vi "Test_LIMS.vi"() -> ()   [LabVIEW 2019]
uses:
  TypeDef/Test.ctl
  TypeDef/Asset.ctl
  TypeDef/Step.ctl
  TypeDef/UpdateLimsTestStepData.ctl
  ByteGSAPIBase.lvclass
panel:
  out "Result Step 2":T1
  in  "instruction_automation":string
  in  "link_automation":string="https://bytelabs.sharepoint.com/:i:/r/sites/RD/Documenti%20condivisi/Knowledge/yoann-siloine-dyaxQ-aoGWY-unsplash.jpg?csf=1&web=1&e=iVCiSf"
  out "Result Step":T2
  in  "duration_hours":dbl
  in  "value":dbl
  in  "step index":i32
  in  "test index":i32
  out "Test Steps List":T3[](array[typedef])
  out "error out":errorcluster
  out "Tests for bench":T5[](array[typedef])
  in  "Postazione/Data":T6
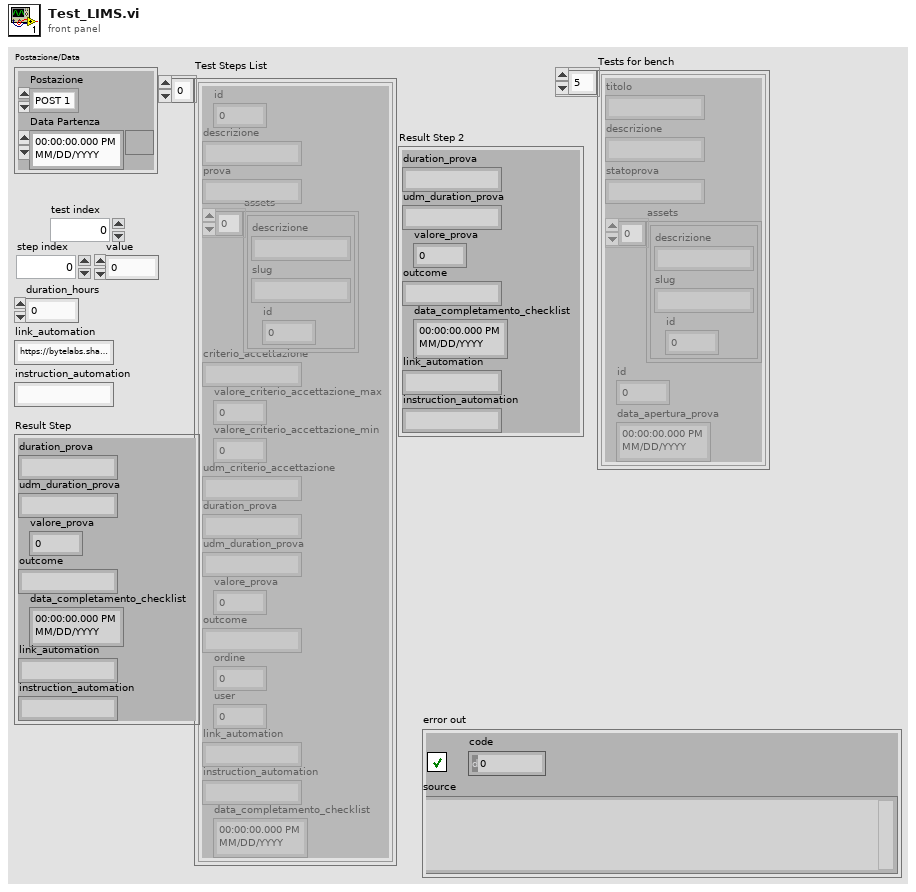
[diagram p1: front panel]
types:
  T1 = typedef "UpdateLimsTestStepData.ctl" = cluster{"duration_prova":string, "udm_duration_prova":string, "valore_prova":dbl, "outcome":string, "data_completamento_checklist":timestamp, "link_automation":string, "instruction_automation":string}
  T2 = cluster{"duration_prova":string, "udm_duration_prova":string, "valore_prova":dbl, "outcome":string, "data_completamento_checklist":timestamp, "link_automation":string, "instruction_automation":string}
  T3 = typedef "ByteGSWebAPI.lvlib/ByteGSAPIBase.lvclass/Step.ctl" = cluster{"id":i32, "descrizione":string, "prova":string, "assets":T4[], "criterio_accettazione":string, "valore_criterio_accettazione_max":dbl, "valore_criterio_accettazione_min":dbl, "udm_criterio_accettazione":string, "duration_prova":string, "udm_duration_prova":string, "valore_prova":dbl, "outcome":string, "ordine":i32, "user":i32, "link_automation":string, "instruction_automation":string, "data_completamento_checklist":timestamp}
  T4 = typedef "ByteGSWebAPI.lvlib/ByteGSAPIBase.lvclass/Asset.ctl" = cluster{"descrizione":string, "slug":string, "id":i32}
  T5 = typedef "ByteGSWebAPI.lvlib/ByteGSAPIBase.lvclass/Test.ctl" = cluster{"titolo":string, "descrizione":string, "statoprova":string, "assets":T4[], "id":i32, "data_apertura_prova":timestamp}
  T6 = cluster{"Postazione":enum16{"POST 1", "POST 2"}, "Data Partenza":timestamp}
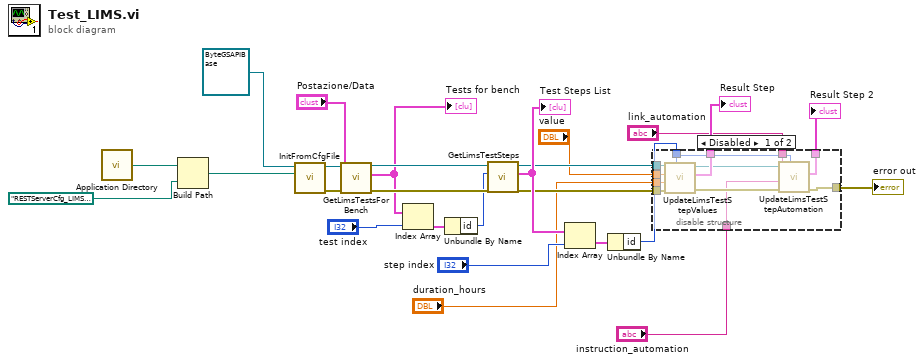
[diagram p0: block diagram]
diagram:
  n1 = call <vilib>:"Application Directory.vi"() -> ("Application Directory"=w26:path)
  n2 = Build Path(base path=w26, name or relative path=path "RESTServerCfg_LIMS.ini") -> (appended path=w23:path)
  n3 = call-dynamic "InitFromCfgFile.vi"("configuration file path"=w23, "ByteGSAPIBase in"=refnum<class "ByteGSAPIBase.lvclass"> refnum) -> ("error out"=w21:errorcluster, "ByteGSAPIBase out"=w22:refnum<class "ByteGSAPIBase.lvclass">)  [unwired: 8 in]
  n4 = call-dynamic "GetLimsTestsForBench.vi"("error in (no error)"=w21, "Data in"="Postazione/Data", "ByteGSAPIBase in"=w22) -> ("error out"=w18:errorcluster, "Tests for bench"=w17:T5[], "ByteGSAPIBase out"=w19:refnum<class "ByteGSAPIBase.lvclass">)  [unwired: 6 in]
  "Tests for bench" <- w17
  n5 = Index Array(array=w17, index="test index") -> (element=w16:T5)
  n6 = Unbundle By Name(w16) -> ("id"=w15:i32)
  n7 = call-dynamic "GetLimsTestSteps.vi"("error in (no error)"=w18, "Test-id"=w15, "ByteGSAPIBase in"=w19) -> ("error out"=w10:errorcluster, "Test Steps List"=w13:T3[], "ByteGSAPIBase out"=w9:refnum<class "ByteGSAPIBase.lvclass">)  [unwired: 6 in]
  "Test Steps List" <- w13
  n8 = Index Array(array=w13, index="step index") -> (element=w11:T3)
  n9 = Unbundle By Name(w11) -> ("id"=w3:i32)
  n10 = disable-structure shown="Disabled" {
    disable-tunnel: w10 -> [w38 _]
    disable-tunnel: w9 -> [w37 _]
    disable-tunnel: "value" -> [w36 _]
    disable-tunnel: "duration_hours" -> [w35 _]
    disable-tunnel: [w34 _] -> w6
    disable-tunnel: "link_automation" -> [w31 _]
    disable-tunnel: "instruction_automation" -> [w30 _]
    disable-tunnel: w3 -> [w29 _]
    disable-tunnel: [w28 _] -> w2
    disable-tunnel: [w27 _] -> w1
    frame Disabled {
      n11 = call-dynamic "UpdateLimsTestStepValues.vi"("step_id"=w29, "error in (no error)"=w38, "duration_hours"=w35, "value"=w36, "ByteGSAPIBase in"=w37) -> ("error out"=w33:errorcluster, "Result Step"=w34:T1, "ByteGSAPIBase out"=w32:refnum<class "ByteGSAPIBase.lvclass">)  [unwired: 4 in]
      n12 = call "UpdateLimsTestStepAutomation.vi"("step_id"=w29, "error in (no error)"=w33, "instruction_automation"=w30, "link_automation"=w31, "ByteGSAPIBase in"=w32) -> ("error out"=w27:errorcluster, "Result Step"=w28:T1)  [unwired: 4 in, 1 out]
    }
    frame Enabled {
    }
  }
  "error out" <- w1
  "Result Step" <- w6
  "Result Step 2" <- w2
